vi "is Running system.vi"(8 "error in (no error)":errorcluster, 10 "Board":u16, 11 "identifier":string) -> (0 "error out":errorcluster, 3 "function return":u32)   [LabVIEW 2015, in "XGL_DPP.lvlib"]
doc: "EXTERN DECLSPEC unsigned int CALL_CONV isRunning_system(const char* identifier, unsigned short Board);"
uses:
  XGL_DPP.lvlib
  XGL_DPP.dll
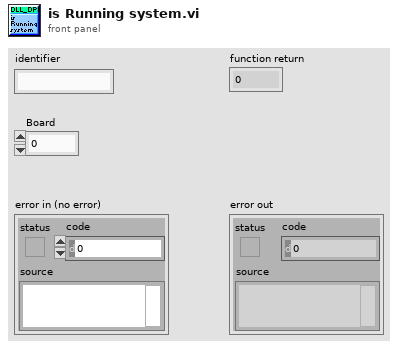
[diagram p1: front panel]
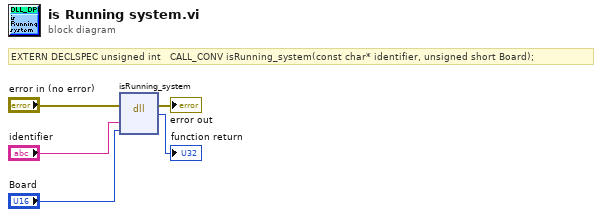
[diagram p0: block diagram]
diagram:
  # "EXTERN DECLSPEC unsigned int   CALL_CONV isRunning_system(const char* identifier, unsigned short Board);"
  n1 = dll-call lib="D:/Users/XRF/Desktop/Dante_acquire4/libs/Dante/XGL_DPP.*" fn="isRunning_system"(error in="error in (no error)", "identifier"="identifier", "Board"="Board") -> (error out=→"error out":errorcluster, "return type"=→"function return":u32)  [unwired: 4 in, 1 out]
